vi "Initialize_WithSerialCommunication.vi"(8 "error in":errorcluster, 10 "Baud Rate":u32(ring)=57600 items=["75"=75, "110"=110, "134"=134, "150"=150, "300"=300, "600"=600, "1200"=1200, "1800"=1800, "2400"=2400, "4800"=4800, "7200"=7200, "9600"=9600, "14400"=14400, "19200"=19200, "28800"=28800, "38400"=38400, "56000"=56000, "57600"=57600, "115200"=115200, "128000"=128000, "230400"=230400], 11 "Comport":refnum<visa-resource-name>="COM20") -> (0 "error out":errorcluster, 1 "FirmataFirmwareVersion":string="v2.5", 2 "FirmataFirmwareName":string="StandardFirmata.ino", 3 "Refnum Out":refnum<vi>, 5 "Connected":bool)   [LabVIEW 2020, in "FirmataClient.lvlib"]
doc: "Initializes the library with a serial comport as the transport method"
uses:
  FirmataClient.lvlib
  Controls/Parameters.ctl
  Controls/TransportParameters.ctl
  Controls/SupportedTransports.ctl
  Controls/FirmataPinCapabilitiesAndAnalogMapping.ctl
  Controls/FirmataPinCapability.ctl
  Controls/FirmataPinModes.ctl
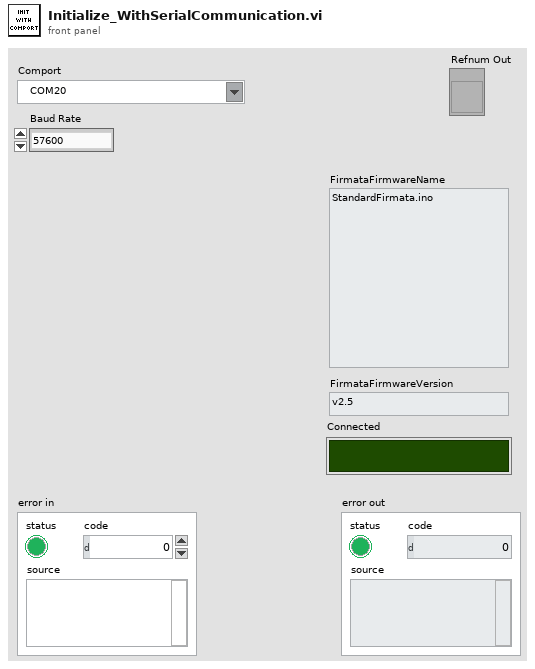
[diagram p1: front panel]
types:
  T1 = typedef "FirmataClient.lvlib/SupportedTransports.ctl" = enum16{"Serial Communication Port"}
  T2 = typedef "FirmataClient.lvlib/Parameters.ctl" = cluster{"Transport Parameters":T3, "Board Capabilities":map{i32, T4}}
  T3 = typedef "FirmataClient.lvlib/TransportParameters.ctl" = cluster{"Serial Communication":cluster{"Comport":refnum<visa-resource-name>, "No Response Timeout Ms":u32, "Response Complete Timeout Ms":u32, "Max Rx Length":u32, "Baud Rate":u32}, "Selected Transport":T1, "Initializer File Path":path, "Cleaner File Path":path, "Transporter File Path":path}
  T4 = typedef "FirmataClient.lvlib/FirmataPinCapabilitiesAndAnalogMapping.ctl" = cluster{"Supported Modes":T5[], "Analog Channel":u8, "Pin Name":string}
  T5 = typedef "FirmataClient.lvlib/FirmataPinCapability.ctl" = cluster{"PinMode":T6, "Resolution":u8}
  T6 = typedef "FirmataClient.lvlib/FirmataPinModes.ctl" = enum16{"DigitalInput", "DigitalOutput", "AnalogInput", "PWM", "Servo", "Shift", "I2C", "OneWire", "Stepper", "Encoder", "Serial", "InputPullup", "Extended.SPI", "Extended.Sonar", "Extended.Tone", "Extended.DHT"}
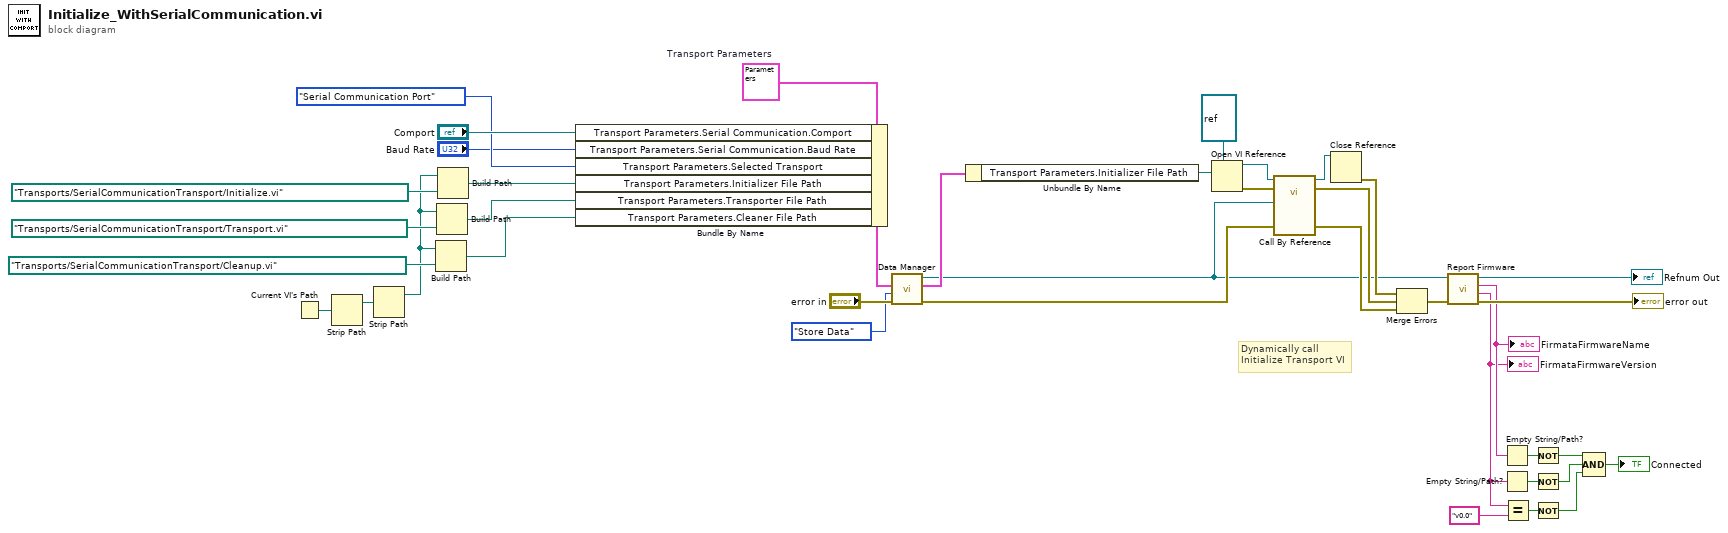
[diagram p0: block diagram]
diagram:
  w33 = T2 {"Transport Parameters"={"Serial Communication"={"Comport"="", "No Response Timeout Ms"=5000, "Response Complete Timeout Ms"=200, "Max Rx Length"=1048, "Baud Rate"=9600}, "Selected Transport"=enum."Serial Communication Port", "Initializer File Path"=path "", "Cleaner File Path"=path "", "Transporter File Path"=path ""}, "Board Capabilities"={}}  # Transport Parameters
  # "Dynamically call\nInitialize Transport VI"
  n1 = Current VI's Path() -> (path=w37:path)
  n2 = Strip Path(path=w37) -> (stripped path=w36:path)  [unwired: 1 out]
  n3 = Strip Path(path=w36) -> (stripped path=w27:path)  [unwired: 1 out]
  n4 = Build Path(base path=w27, name or relative path=path "Transports/SerialCommunicationTransport/Cleanup.vi" ("Serial Communication.Transporter File Path")) -> (appended path=w25:path)
  n5 = Build Path(base path=w27, name or relative path=path "Transports/SerialCommunicationTransport/Transport.vi" ("Serial Communication.Transporter File Path")) -> (appended path=w26:path)
  n6 = Build Path(base path=w27, name or relative path=path "Transports/SerialCommunicationTransport/Initialize.vi" ("Serial Communication.Transporter File Path")) -> (appended path=w34:path)
  n7 = Bundle By Name(cluster=w33, "Transport Parameters.Serial Communication.Comport"="Comport", "Transport Parameters.Serial Communication.Baud Rate"="Baud Rate", "Transport Parameters.Selected Transport"=SupportedTransports."Serial Communication Port" ("Selected Transport"), "Transport Parameters.Initializer File Path"=w34, "Transport Parameters.Transporter File Path"=w26, "Transport Parameters.Cleaner File Path"=w25) -> (w31:T2)
  n8 = call "Data Manager.vi"("error in (no error)"="error in", "Mode"=enum16{"Store Data", "Get Data", "Cleanup"}."Store Data", "Data In"=w31) -> ("error out"=w18:errorcluster, "Data Out"=w20:T2, "Refnum Out"=w1:refnum<vi>)  [unwired: 6 in]
  n9 = Unbundle By Name(w20) -> ("Transport Parameters.Initializer File Path"=w19:path)
  n10 = Open VI Reference(type specifier VI Refnum (for type only)=refnum<vi> refnum, vi path=w19) -> (vi reference=w22:refnum<vi>, error out=w23:errorcluster)  [unwired: 4 in]
  n11 = call-by-ref "?"(reference=w22, error in=w23, "error in"=w18, "Refnum In"=w1) -> (reference out=w21:refnum<vi>, error out=w15:errorcluster, 0:"error out"=w16:errorcluster)  [unwired: 8 in, 1 out]
  n12 = Close Reference(reference=w21) -> (error out=w17:errorcluster)  [unwired: 1 in]
  n13 = Merge Errors(w17, w15, w16) -> (w14:errorcluster)
  n14 = call "Report Firmware.vi"("error in (no error)"=w14, "Refnum In"=w1) -> ("error out"=→"error out":errorcluster, "FirmataFirmwareVersion"=w6:string, "FirmataFirmwareName"=w11:string, "Refnum Out"=→"Refnum Out":refnum<vi>)  [unwired: 6 in]
  "FirmataFirmwareName" <- w11
  "FirmataFirmwareVersion" <- w6
  n15 = Empty String/Path?(string/path=w11) -> (empty?=w10:bool)
  n16 = Empty String/Path?(string/path=w6) -> (empty?=w9:bool)
  n17 = Equal?(x=w6, y="v0.0") -> (x = y?=w5:bool)
  n18 = Not(x=w10) -> (.not. x?=w8:bool)
  n19 = Not(x=w9) -> (.not. x?=w7:bool)
  n20 = Not(x=w5) -> (.not. x?=w4:bool)
  n21 = Compound Arithmetic op=AND(w8, w7, w4) -> (→"Connected":bool)
